vi "Main.vi"(11 "Module Admin":refnum<class "Delacor_lib_QMH_Module Admin.lvclass">) -> ()   [LabVIEW 2020, in "Stock.lvlib"]
doc: "This template is based off of the Queued Message Handler design pattern and the Queued Message Handler project template that ships with LabVIEW.\n\nThe main difference is that the queue is private to this module and communication between modules is performed via Broadcast and Request events.\n\nRequest events are wrapped in public API methods and are handled in the Event Handling Loop (EHL) of this VI. Any module can register for Broadcast events sent by this module. The EHL generates messages based on user interface actions.\n\nThe Message Handling Loop (MHL) processes messages generated by the EHL, or by other messages. The messages are string values, so new messages can be added easily to the Message Cases case structure in the MHL. Each message cluster can also provide an optional value for Message Data, which is a variant that can be converted to whatever message-specific data is required.\n_____\nBased on Delacor QMH Project Template 5.0.0.82."
uses:
  Stock.lvlib
  <vilib>/Delacor/Delacor QMH/Libraries/Module Admin_class/Delacor_lib_QMH_Module Admin.lvclass
  Module Data--cluster.ctl
  <vilib>/Delacor/Delacor QMH/Libraries/Message Queue_class/Delacor_lib_QMH_Message Queue.lvclass/Delacor_lib_QMH_Message Queue.ctl
  Stop Argument--cluster.ctl
  <vilib>/Delacor/Delacor QMH/Libraries/Module Admin_class/Delacor_lib_QMH_Module Admin.lvclass/Delacor_lib_QMH_Module Admin.ctl
  Check Product Availability Argument--cluster.ctl
  Check Product Availability (Reply Payload)--cluster.ctl
  Extract Product Argument--cluster.ctl
  <vilib>/Utility/miscctls.llb/LVPointTypeDef.ctl
  <vilib>/Delacor/Delacor QMH/Libraries/Message Queue_class/Delacor_lib_QMH_Enqueue Message (Single).vi
  <vilib>/Delacor/Delacor QMH/Libraries/Module Admin_class/Delacor_lib_QMH_Get External Launch.vi
  <vilib>/Utility/error.llb/Error Cluster From Error Code.vi
  <vilib>/ErrorRing/Error Ring.xnode
  <vilib>/Delacor/Delacor QMH/Libraries/Message Queue_class/Delacor_lib_QMH_Message Queue.lvclass
panel:
  in  "Products":T1(array[cluster])=[{"Product name"="Coke", "Quantity"=10.0, "Price"=5.0}, {"Product name"="Sprite", "Quantity"=10.0, "Price"=4.5}, {"Product name"="Orange Juice", "Quantity"=10.0, "Price"=6.0}, {"Product name"="Regular water", "Quantity"=10.0, "Price"=3.5}, {"Product name"="Sparking water", "Quantity"=10.0, "Price"=3.5}]
  in  "Simulate MHL Error":bool
  in  "Simulate EHL Error":bool
  out "error out":errorcluster
  out "Status":string
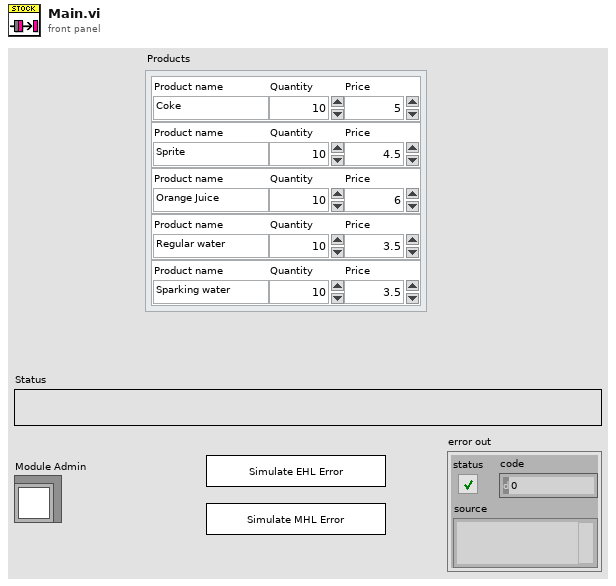
[diagram p1: front panel]
types:
  T1 = cluster{"Product name":string, "Quantity":dbl, "Price":dbl}[]
  T2 = typedef "Stock.lvlib/Request Events--cluster.ctl" = cluster{"Stop Module":refnum<user-event>, "Show Panel":refnum<user-event>, "Hide Panel":refnum<user-event>, "Get Module Execution Status":refnum<user-event>, "Show Diagram":refnum<user-event>, "Check Product Availability":refnum<user-event>, "Extract Product":refnum<user-event>}
  T3 = typedef "Stock.lvlib/Module Data--cluster.ctl" = cluster{"Status":string, "Map":map{string, cluster{"Product name":string, "Quantity":dbl, "Price":dbl}}}
  T4 = enum32{"invalid lock state", "Not Locked", "Locked (No Password)", "Password-protected"}
  T5 = typedef "Stock.lvlib/Stop Argument--cluster.ctl" = cluster{"Origin":string, "Exit via Stop Module Req?":bool, "Wait for Module to stop?":bool}
  T6 = typedef "Stock.lvlib/Check Product Availability Argument--cluster.ctl" = cluster{"Product name":string, "Wait Notifier":refnum<notifier>, "wait for reply":bool}
  T7 = typedef "Stock.lvlib/Extract Product Argument--cluster.ctl" = cluster{"Product name":string}
  T8 = typedef "LVPointTypeDef.ctl" = cluster{"Horizontal":i16, "Vertical":i16}
  T9 = enum32{"Invalid", "Standard", "Closed", "Hidden", "Minimized", "Maximized"}
  T10 = typedef "Stock.lvlib/Check Product Availability (Reply Payload)--cluster.ctl" = cluster{"Product in stock":bool, "Check Product Availability_error":errorcluster}
  T11 = map{string, cluster{"Product name":string, "Quantity":dbl, "Price":dbl}}
  T12 = cluster{"Product name":string, "Quantity":dbl, "Price":dbl}
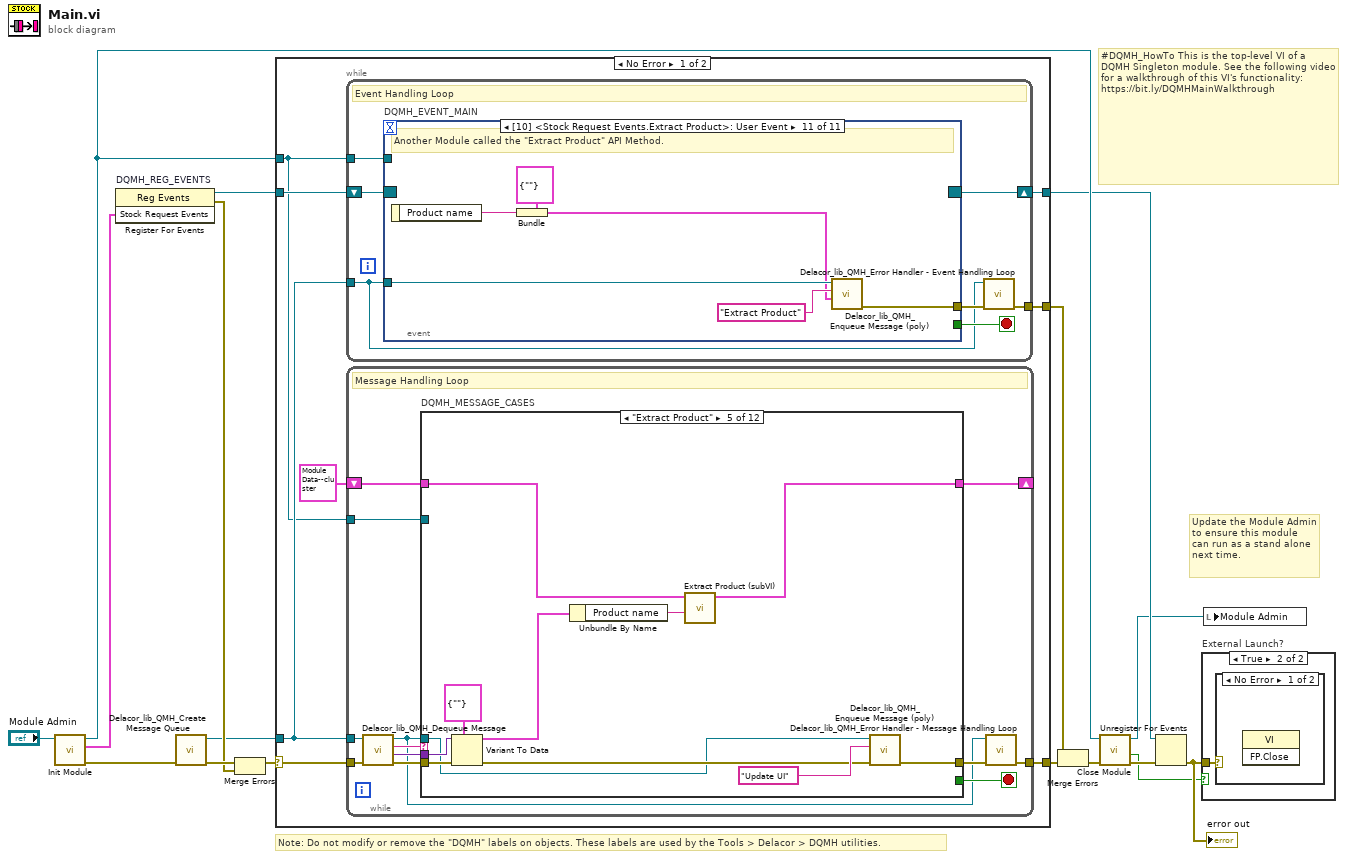
[diagram p0: block diagram]
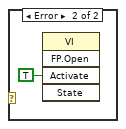
[diagram p3: hidden frame]
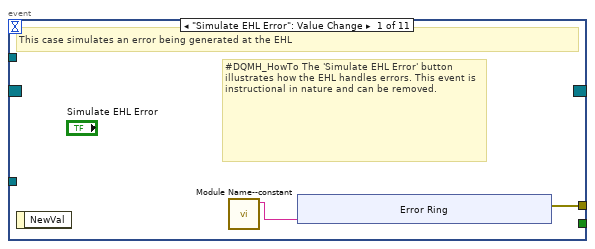
[diagram p4: hidden frame]
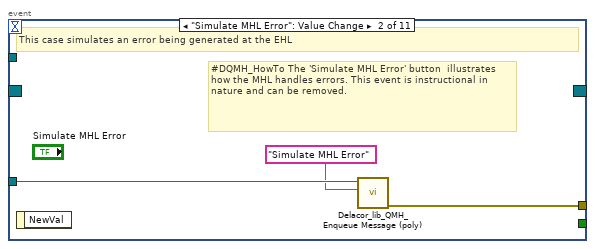
[diagram p5: hidden frame]
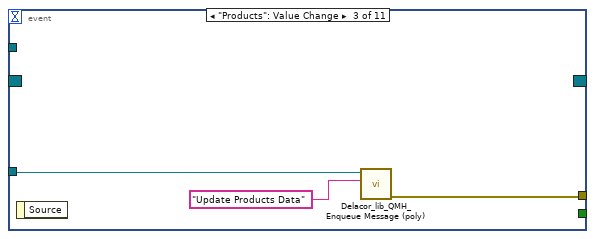
[diagram p6: hidden frame]
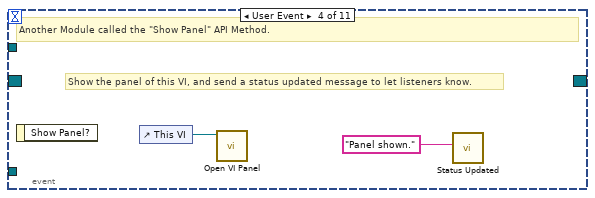
[diagram p7: hidden frame]
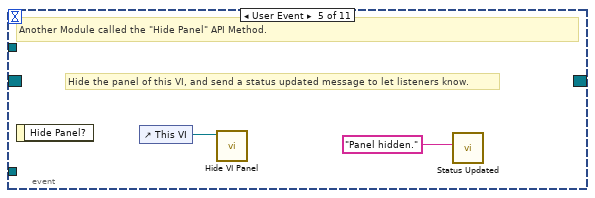
[diagram p8: hidden frame]
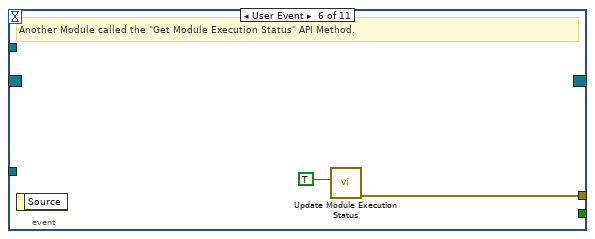
[diagram p9: hidden frame]
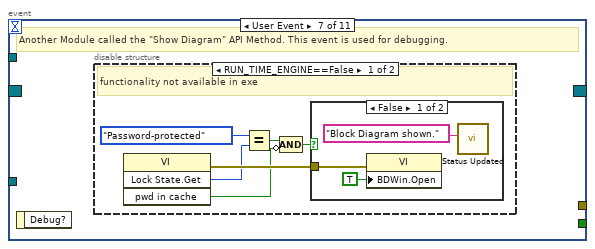
[diagram p10: hidden frame]
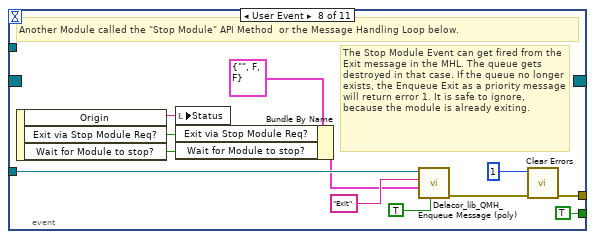
[diagram p13: hidden frame]
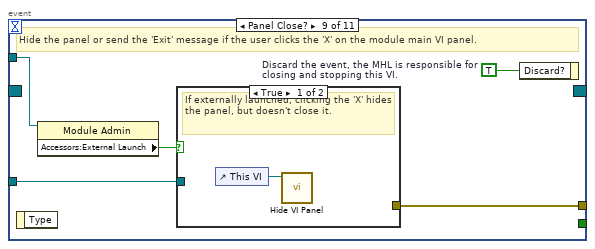
[diagram p14: hidden frame]
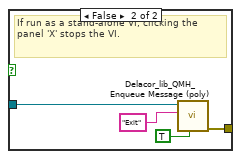
[diagram p15: hidden frame]
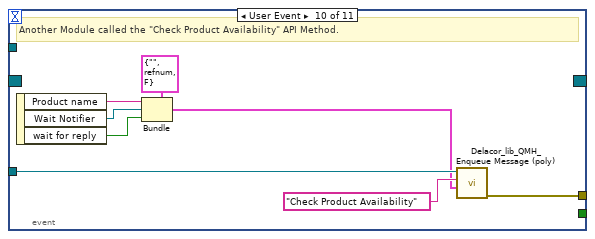
[diagram p16: hidden frame]
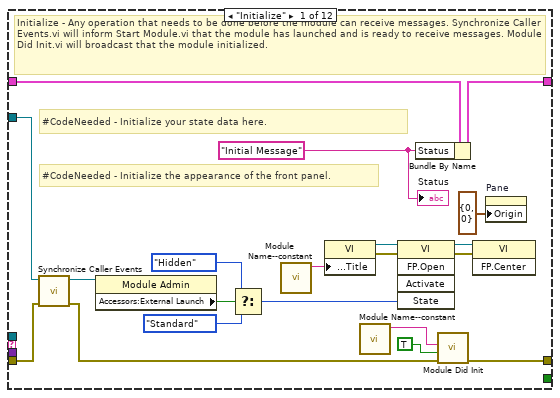
[diagram p17: hidden frame]
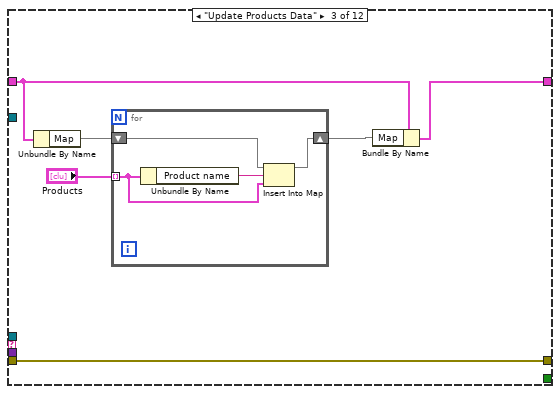
[diagram p19: hidden frame]
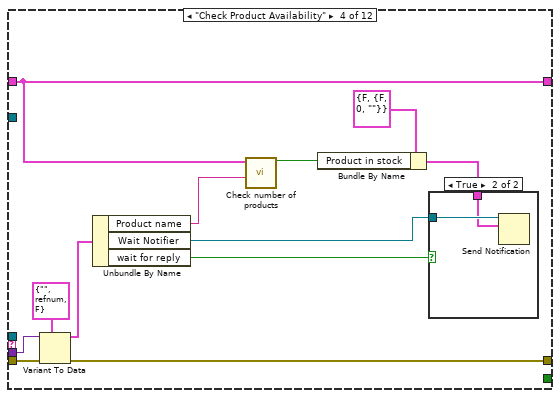
[diagram p20: hidden frame]
diagram:
  # "#DQMH_HowTo This is the top-level VI of a DQMH Singleton module. See the following video for a walkthrough of this VI's functionality: https://bit.ly/DQMHMainWalkthrough"
  # "Note: Do not modify or remove the \"DQMH\" labels on objects. These labels are used by the Tools > Delacor > DQMH utilities."
  # "Update the Module Admin to ensure this module can run as a stand alone next time."
  n1 = call "Init Module.vi"("Singleton Module Admin in"="Module Admin") -> ("error out"=w16:errorcluster, "Stock Request Events"=w5:T2, "Singleton Module Admin out"=w8:refnum<class "Delacor_lib_QMH_Module Admin.lvclass">)  [unwired: 8 in]
  n2 = register-events "DQMH_REG_EVENTS"(w5) -> (reference out=w6:refnum<event-registration>, error out=w9:errorcluster)  [unwired: 2 in]
  n3 = call <vilib>:"Delacor_lib_QMH_Create Message Queue.vi"("error in (no error)"=w16) -> ("error out"=w11:errorcluster, "Message Queue"=w4:refnum<class "Delacor_lib_QMH_Message Queue.lvclass">)  [unwired: 9 in]
  n4 = Merge Errors(w11, w9) -> (w10:errorcluster)
  n5 = case shown="No Error" w10 {
    selector: w10 -> [w23 w239]
    tunnel: [w25 w238] -> w17
    tunnel: [w22 w244] -> w7
    tunnel: w6 -> [w20 w244]
    tunnel: w4 -> [w19 w237]
    tunnel: [w24 _] -> w14
    tunnel: w8 -> [w18 w240]
    frame No Error {
      n6 = while {
        tunnel: w19 -> [w26]
        shift-right: [w29] -> w22
        shift-left: w20 -> [w30]
        tunnel: [w31] -> w24
        tunnel: w18 -> [w27]
        stop <- w28 stop-if-true
        # "Event Handling Loop"
        n7 = event "DQMH_EVENT_MAIN" shown="[10] <Stock Request Events.Extract Product>: User Event" {
          selector: w30 -> [_ _ _ _ _ _ _ _ _ _ _]
          dyn-events: [_ _ _ _ _ _ _ _ _ _ _] -> w29
          timeout: _ -> [_ _ _ _ _ _ _ _ _ _ _]
          tunnel: [_ _ _ _ _ _ _ TRUE ("Discard?") _ _ _] -> w28
          tunnel: w26 -> [_ w43 w46 _ _ _ _ w70 w77 w92 w98]
          tunnel: [w34 w44 w45 _ _ w53 _ w73 w79 w85 w93] -> w32
          tunnel: w27 -> [_ _ _ _ _ _ _ _ w76 _ _]
          event "Simulate EHL Error": Value Change {
            # "#DQMH_HowTo The 'Simulate EHL Error' button  illustrates how the EHL handles errors. This event is instructional in nature and can be removed."
            # "This case simulates an error being generated at the EHL"
            n8 = event-data() -> ()  [unwired: 1 in, 1 out]
            n9 = call "Module Name--constant.vi"() -> ("Module Name"=w33:string)  [unwired: 11 in]
            n10 = xnode "Error Ring"("parameter 0"=w33) -> ("error out"=w34:errorcluster)
          }
          event "Simulate MHL Error": Value Change {
            # "#DQMH_HowTo The 'Simulate MHL Error' button  illustrates how the MHL handles errors. This event is instructional in nature and can be removed."
            # "This case simulates an error being generated at the EHL"
            n11 = event-data() -> ()  [unwired: 1 in, 1 out]
            n12 = call-poly <vilib>:"Delacor_lib_QMH_Enqueue Message (poly).vi"("Message"="Simulate MHL Error", "Message Queue in"=w43) -> ("error out"=w44:errorcluster)  [unwired: 8 in, 1 out]
          }
          event "Products": Value Change {
            n13 = event-data() -> ()  [unwired: 1 in, 1 out]
            n14 = call-poly <vilib>:"Delacor_lib_QMH_Enqueue Message (poly).vi"("Message"="Update Products Data", "Message Queue in"=w46) -> ("error out"=w45:errorcluster)  [unwired: 8 in, 1 out]
          }
          event User Event {
            # "Show the panel of this VI, and send a status updated message to let listeners know."
            # "Another Module called the \"Show Panel\" API Method."
            n15 = event-data() -> ()  [unwired: 1 in, 1 out]
            n16 = control-ref of="This VI"() -> (w49:refnum<vi>)
            n17 = call "Open VI Panel.vi"("VI"=w49) -> ()  [unwired: 10 in, 1 out]
            n18 = call "Status Updated.vi"("Status"="Panel shown." ("format string")) -> ()  [unwired: 10 in, 1 out]
          }
          event User Event {
            # "Hide the panel of this VI, and send a status updated message to let listeners know."
            # "Another Module called the \"Hide Panel\" API Method."
            n19 = event-data() -> ()  [unwired: 1 in, 1 out]
            n20 = control-ref of="This VI"() -> (w51:refnum<vi>)
            n21 = call "Hide VI Panel.vi"("VI"=w51) -> ()  [unwired: 10 in, 1 out]
            n22 = call "Status Updated.vi"("Status"="Panel hidden." ("format string")) -> ()  [unwired: 10 in, 1 out]
          }
          event User Event {
            # "Another Module called the \"Get Module Execution Status\" API Method."
            n23 = event-data() -> ()  [unwired: 1 in, 1 out]
            n24 = call "Update Module Execution Status.vi"("Running?"=TRUE) -> ("error out"=w53:errorcluster)  [unwired: 10 in]
          }
          event User Event {
            # "Another Module called the \"Show Diagram\" API Method. This event is used for debugging."
            n25 = event-data() -> ()  [unwired: 1 in, 1 out]
            n26 = disable-structure shown="RUN_TIME_ENGINE==False" {
              frame condition #0 (active) {
                # "functionality not available in exe"
                n27 = invoke class="VI" method="Lock State.Get"() -> (error out=w59:errorcluster, "Get Lock State"=w58:T4, "pwd in cache"=w55:bool)  [unwired: 4 in, 1 out]
                n28 = Equal?(x=T4."Password-protected", y=w58) -> (x = y?=w56:bool)
                n29 = Compound Arithmetic op=AND(w56, invert w55) -> (w54:bool)
                n30 = case shown="False" w54 {
                  tunnel: w59 -> [w62 _]
                  frame False {
                    n31 = property class="VI"(error in=w62, "BDWin.Open"=TRUE ("Block Diagram Window:Open")) -> ()  [unwired: 1 in, 2 out]
                    n32 = call "Status Updated.vi"("Status"="Block Diagram shown." ("format string")) -> ()  [unwired: 10 in, 1 out]
                  }
                  frame True {
                    # "Password-protected VI, and the password is not in the cache. Do not show the diagram."
                  }
                }
              }
              frame condition #1 {
              }
            }
          }
          event User Event {
            # "The Stop Module Event can get fired from the Exit message in the MHL. The queue gets destroyed in that case. If the queue no longer exists, the Enqueue Exit as a priority message will return error 1. It is safe to ignore, because the module is already exiting."
            # "Another Module called the \"Stop Module\" API Method  or the Message Handling Loop below."
            n33 = event-data() -> ("Origin"=w69:string, "Exit via Stop Module Req?"=w65:bool, "Wait for Module to stop?"=w64:bool)  [unwired: 1 in]
            n34 = local write "Status"(w69) -> ()
            n35 = Bundle By Name(cluster=T5 {"Origin"="", "Exit via Stop Module Req?"=FALSE, "Wait for Module to stop?"=FALSE} ("Stop Argument"), "Exit via Stop Module Req?"=w65, "Wait for Module to stop?"=w64) -> (w63:T5)
            n36 = call-poly <vilib>:"Delacor_lib_QMH_Enqueue Message (poly).vi"("Priority Message? (F)"=TRUE, "Message Data"=w63, "Message"="Exit", "Message Queue in"=w70) -> ("error out"=w74:errorcluster)  [unwired: 6 in, 1 out]
            n37 = call <vilib>:"Clear Errors.vi"("error in (no error)"=w74, "specific error code to clear (0: all)"=1) -> ("error out"=w73:errorcluster)  [unwired: 4 in, 1 out]
          }
          event Panel Close? {
            w78 = TRUE  # Discard the event, the MHL is responsible for closing and stopping this VI.
            # "Hide the panel or send the 'Exit' message if the user clicks the 'X' on the module main VI panel."
            n38 = event-data() -> ()  [unwired: 1 in, 1 out]
            n39 = property class="Module Admin"(reference=w76) -> ("Accessors:External Launch"=w75:bool)  [unwired: 1 in, 2 out]
            n40 = case shown="True" w75 {
              tunnel: w77 -> [_ w83]
              tunnel: [_ w84] -> w79
              frame True {
                # "If externally launched, clicking the 'X' hides the panel, but doesn't close it."
                n41 = control-ref of="This VI"() -> (w80:refnum<vi>)
                n42 = call "Hide VI Panel.vi"("VI"=w80) -> ()  [unwired: 10 in, 1 out]
              }
              frame False {
                # "If run as a stand-alone VI, clicking the panel 'X' stops the VI."
                n43 = call-poly <vilib>:"Delacor_lib_QMH_Enqueue Message (poly).vi"("Priority Message? (F)"=TRUE, "Message"="Exit", "Message Queue in"=w83) -> ("error out"=w84:errorcluster)  [unwired: 7 in, 1 out]
              }
            }
            n44 = event-data("Discard?"=w78) -> ()  [unwired: 1 in, 1 out]
          }
          event User Event {
            # "Another Module called the \"Check Product Availability\" API Method."
            n45 = event-data() -> ("Product name"=w88:string, "Wait Notifier"=w87:refnum<notifier>, "wait for reply"=w86:bool)  [unwired: 1 in]
            n46 = Bundle(cluster=T6 {"Product name"="", "Wait Notifier"=refnum, "wait for reply"=FALSE} ("Check Product Availability Argument"), "Product name"=w88, "Wait Notifier"=w87, "wait for reply"=w86) -> (w89:T6)
            n47 = call-poly <vilib>:"Delacor_lib_QMH_Enqueue Message (poly).vi"("Message Data"=w89, "Message"="Check Product Availability", "Message Queue in"=w92) -> ("error out"=w85:errorcluster)  [unwired: 7 in, 1 out]
          }
          event User Event {
            # "Another Module called the \"Extract Product\" API Method."
            n48 = event-data() -> ("Product name"=w94:string)  [unwired: 1 in]
            n49 = Bundle(cluster=T7 {"Product name"=""} ("Extract Product Argument"), "Product name"=w94) -> (w95:T7)
            n50 = call-poly <vilib>:"Delacor_lib_QMH_Enqueue Message (poly).vi"("Message Data"=w95, "Message"="Extract Product", "Message Queue in"=w98) -> ("error out"=w93:errorcluster)  [unwired: 7 in, 1 out]
          }
        }
        n51 = call-dynamic "Delacor_lib_QMH_Error Handler - Event Handling Loop.vi"("error in (no error)"=w32, "Message Queue in"=w26) -> ("dup error in"=w31:errorcluster)  [unwired: 8 in, 1 out]
      }
      n52 = while {
        tunnel: w19 -> [w101]
        shift-right: [w105] -> _
        shift-left: T3 {"Status"="", "Map"={}} ("Data Cluster") -> [w106]
        tunnel: w23 -> [w109]
        tunnel: [w107] -> w25
        tunnel: w18 -> [w99]
        stop <- w104 stop-if-true
        # "Message Handling Loop"
        n53 = call-dynamic "Delacor_lib_QMH_Dequeue Message.vi"("error in (no error)"=w109, "Message Queue in"=w101) -> ("error out"=w108:errorcluster, "Message Data"=w102:variant, "Message"=w103:string, "Message Queue out"=w100:refnum<class "Delacor_lib_QMH_Message Queue.lvclass">)  [unwired: 6 in]
        n54 = case "DQMH_MESSAGE_CASES" shown="\"Extract Product\"" w103 {
          selector: w103 -> [_ _ _ _ _ _ _ _ _ _ _ w224]
          tunnel: w100 -> [_ _ _ _ w157 _ _ _ _ w194 w216 _]
          tunnel: w108 -> [w128 w132 w138 w154 w167 w171 w176 w178 w183 w201 w222 w226]
          tunnel: [w126 w132 w138 w143 w158 w171 w175 w178 w182 w197 w219 w227] -> w110
          tunnel: w106 -> [w117 w131 w134 w146 w163 w170 w174 w177 w180 w196 w215 w225]
          tunnel: [w116 w131 w137 w146 w162 w170 w174 w177 w180 w196 w215 w225] -> w105
          tunnel: [_ _ _ _ _ _ _ _ _ _ w214 _] -> w104
          tunnel: w102 -> [_ _ _ w153 w166 _ _ _ _ w195 w213 _]
          tunnel: w99 -> [w118 _ _ _ _ _ _ _ _ w193 w208 _]
          frame "Initialize" {
            w111 = "Initial Message" ("Initial Message")
            # "#CodeNeeded - Initialize the appearance of the front panel."
            # "#CodeNeeded - Initialize your state data here."
            # "Initialize - Any operation that needs to be done before the module can receive messages. Synchronize Caller Events.vi will inform Start Module.vi that the module has launched and is ready to receive messages. Module Did Init.vi will broadcast that the module initialized."
            n55 = call "Synchronize Caller Events.vi"("error in (no error)"=w128, "Singleton Module Admin in"=w118) -> ("error out"=w127:errorcluster, "Singleton Module Admin out"=w113:refnum<class "Delacor_lib_QMH_Module Admin.lvclass">)  [unwired: 8 in]
            n56 = property class="Module Admin"(reference=w113) -> ("Accessors:External Launch"=w122:bool)  [unwired: 1 in, 2 out]
            n57 = Select(t=T9."Hidden" ("State"), s=w122, f=T9."Standard" ("State")) -> (s? t:f=w119:T9)
            n58 = call "Module Name--constant.vi"() -> ("Module Name"=w125:string)  [unwired: 11 in]
            n59 = property class="VI"("Front Panel.Title"=w125) -> (reference out=w124:refnum<vi>, error out=w130:errorcluster)  [unwired: 2 in]
            n60 = call "Module Name--constant.vi"() -> ("Module Name"=w114:string)  [unwired: 11 in]
            n61 = invoke class="VI" method="FP.Open"(reference=w124, error in=w130, "State"=w119) -> (reference out=w123:refnum<vi>, error out=w129:errorcluster)  [unwired: 2 in, 3 out]
            n62 = Bundle By Name(cluster=w117, "Status"=w111) -> (w116:T3)
            n63 = call "Module Did Init.vi"("error in (no error)"=w127, "Initialized?"=TRUE, "Origin"=w114) -> ("error out"=w126:errorcluster)  [unwired: 8 in]
            n64 = invoke class="VI" method="FP.Center"(reference=w123, error in=w129) -> ()  [unwired: 1 in, 3 out]
            n65 = property on="Pane" class="Pane"("Origin"=T8 {"Horizontal"=0, "Vertical"=0}) -> ()  [unwired: 2 in, 2 out]
            "Status" <- w111
          }
          frame "--- Module Specific ---" {
            # "Separator -- The following cases handle messages specific to this Module."
          }
          frame "Update Products Data" {
            n66 = Unbundle By Name(w134) -> ("Map"=w135:T11)
            n67 = for {
              tunnel: "Products" -> [w141] mode=indexing
              shift-right: [w139] -> w133
              shift-left: w135 -> [w140]
              n68 = Unbundle By Name(w141) -> ("Product name"=w142:string)
              n69 = Insert Into Map(map in=w140, key=w142, value=w141) -> (map out=w139:T11)  [unwired: 2 out]
            }
            n70 = Bundle By Name(cluster=w134, "Map"=w133) -> (w137:T3)
          }
          frame "Check Product Availability" {
            n71 = Variant To Data(error in=w154, type=T6 {"Product name"="", "Wait Notifier"=refnum, "wait for reply"=FALSE} ("Check Product Availability Argument"), Variant=w153) -> (data=w151:T6, error out=w143:errorcluster)
            n72 = Unbundle By Name(w151) -> ("Product name"=w145:string, "Wait Notifier"=w150:refnum<notifier>, "wait for reply"=w149:bool)
            n73 = call "Check number of products.vi"("Product name"=w145, "Data Cluster"=w146) -> ("Product Available"=w144:bool)  [unwired: 9 in]
            n74 = Bundle By Name(cluster=T10 {"Product in stock"=FALSE, "Check Product Availability_error"={"status"=FALSE, "code"=0, "source"=""}} ("Check Product Availability (Reply Payload)"), "Product in stock"=w144) -> (w148:T10)
            n75 = case shown="True" w149 {
              tunnel: w150 -> [_ w156]
              tunnel: w148 -> [_ w155]
              frame False {
              }
              frame True {
                n76 = Send Notification(notification=w155, notifier=w156) -> ()  [unwired: 1 in, 2 out]
              }
            }
          }
          frame "Extract Product" {
            n77 = Variant To Data(error in=w167, type=T7 {"Product name"=""} ("Extract Product Argument"), Variant=w166) -> (data=w164:T7, error out=w159:errorcluster)
            n78 = Unbundle By Name(w164) -> ("Product name"=w161:string)
            n79 = call "Extract Product (subVI).vi"("Product name"=w161, "Data Cluster"=w163) -> ("Data cluster output"=w162:T3)  [unwired: 9 in]
            n80 = call-poly <vilib>:"Delacor_lib_QMH_Enqueue Message (poly).vi"("error in (no error)"=w159, "Message"="Update UI", "Message Queue in"=w157) -> ("error out"=w158:errorcluster)  [unwired: 7 in, 1 out]
          }
          frame "Update UI" {
            n81 = Unbundle By Name(w170) -> ("Map"=w169:T11)
            n82 = for {
              tunnel: w169 -> [w173] mode=indexing
              tunnel: [w172] -> w168 mode=indexing
              n83 = Unbundle By Name(w173) -> ("Cluster"=w172:T12)
            }
            n84 = local write "Products"(w168) -> ()
          }
          frame "---Copy This Frame---" {
            # "Duplicate this frame when creating new messages.  Change this comment in the duplicated frame to describe this message."
            n85 = Merge Errors(w176) -> (w175:errorcluster)
          }
          frame "--- Exit and Error Handling---" {
            # "Separator - The following cases handle errors and exit messages."
          }
          frame "Simulate MHL Error" {
            # "#DQMH_HowTo The 'Simulate MHL Error' button  illustrates how the MHL handles errors. This event is instructional in nature and can be removed."
            # "Simulate an error occurring at the MHL"
            n86 = call "Module Name--constant.vi"() -> ("Module Name"=w179:string)  [unwired: 11 in]
            n87 = xnode "Error Ring"("parameter 0"=w179) -> ("error out"=w181:errorcluster)
            n88 = Merge Errors(w183, w181) -> (w182:errorcluster)
          }
          frame "Error" {
            # "#CodeRecommended - If you ever change the name of this \"Error\" message, you'll need to update the name in the Check Loop Error.vi as well."
            # "#CodeRecommended - If the module is running in standalone mode (External Launch = FALSE), this code will pop up an error dialog and call the 'Exit' message if an error occurs. Add more fine-grained error handling here."
            # "Error - Check the error message data and respond accordingly. This message is sent by the \"Error Handler\" VIs at the end of each loop in this application."
            n89 = property class="Module Admin"(reference=w193) -> ("Accessors:External Launch"=w192:bool)  [unwired: 1 in, 2 out]
            n90 = Variant To Data(error in=w201, type=errorcluster {"status"=FALSE, "code"=0, "source"=""} ("error constant"), Variant=w195) -> (data=w202:errorcluster, error out=w199:errorcluster)
            n91 = call "Module Name--constant.vi"() -> ("Module Name"=w191:string)  [unwired: 11 in]
            n92 = call "Error Reported.vi"("Additional Information"=w191, "Error"=w202) -> ()  [unwired: 9 in, 1 out]
            n93 = case shown="False" w192 {
              tunnel: [w207 _] -> w198
              tunnel: w194 -> [w205 _]
              tunnel: w202 -> [w206 _]
              frame False {
                # "If the module is running standalone, then pop up an error dialog and call the \"Exit\" message."
                n94 = call <vilib>:"Simple Error Handler.vi"("error in (no error)"=w206) -> ()  [unwired: 4 in, 5 out]
                n95 = call-poly <vilib>:"Delacor_lib_QMH_Enqueue Message (poly).vi"("Priority Message? (F)"=TRUE, "Message"="Exit", "Message Queue in"=w205) -> ("error out"=w207:errorcluster)  [unwired: 7 in, 1 out]
              }
              frame True {
                # "If the module was launched externally, calling the Error Reported broadcast VI is the only action performed by the \"Error\" message. The module's caller can then process the error appropriately."
              }
            }
            n96 = Merge Errors(w199, w198) -> (w197:errorcluster)
            n97 = local write "error out"(w197) -> ()
          }
          frame "Exit" {
            w212 = 91  # 91: not all Exit messages will have an argument
            w214 = TRUE  # Stop the VI
            # "Release the message queue reference"
            # "#CodeNeeded - Add any required cleanup code here"
            # "Exit - Exit the application."
            n98 = Variant To Data(error in=w222, type=T5 {"Origin"="", "Exit via Stop Module Req?"=FALSE, "Wait for Module to stop?"=FALSE} ("Stop Argument"), Variant=w213) -> (data=w210:T5, error out=w218:errorcluster)
            n99 = call <vilib>:"Clear Errors.vi"("error in (no error)"=w218, "specific error code to clear (0: all)"=w212) -> ("error out"=w221:errorcluster)  [unwired: 4 in, 1 out]
            n100 = control-ref of="This VI"() -> (w209:refnum<vi>)
            n101 = call-dynamic "Delacor_lib_QMH_Release Message Queue.vi"("error in (no error)"=w221, "Message Queue"=w216) -> ("error out"=w220:errorcluster)  [unwired: 9 in]
            n102 = call "Handle Exit.vi"("Stop Argument"=w210, "Admin in"=w208, "VI reference"=w209) -> ("error out"=w217:errorcluster)  [unwired: 7 in, 1 out]
            n103 = Merge Errors(w220, w217) -> (w219:errorcluster)
          }
          frame Default {
            # "'Default' case only runs if there is a message that isn't defined in any of the other cases.  Output a programming error."
            n104 = call "Module Name--constant.vi"() -> ("Module Name"=w223:string)  [unwired: 11 in]
            n105 = xnode "Error Ring"("parameter 0"=w224, "parameter 1"=w223) -> ("error out"=w228:errorcluster)
            n106 = Merge Errors(w226, w228) -> (w227:errorcluster)
          }
        }
        n107 = call-dynamic "Delacor_lib_QMH_Error Handler - Message Handling Loop.vi"("error in (no error)"=w110, "Message Queue in"=w100) -> ("dup error in"=w107:errorcluster)  [unwired: 8 in, 1 out]
      }
    }
    frame Error {
      # "Synchronize Caller Events.vi will inform Start Module.vi that the module has launched and will let the code calling Start Module.vi register for broadcasts and would permit the caller receive the broadcast that an error occurred at launch time."
      n108 = call-dynamic "Delacor_lib_QMH_Release Message Queue.vi"("error in (no error)"=w239, "Message Queue"=w237) -> ("error out"=w238:errorcluster)  [unwired: 9 in]
      n109 = call "Synchronize Caller Events.vi"("Singleton Module Admin in"=w240) -> ("error out"=w245:errorcluster)  [unwired: 9 in, 1 out]
      n110 = call "Module Name--constant.vi"() -> ("Module Name"=w243:string)  [unwired: 11 in]
      n111 = Format Into String(format string="An error occurred during initialization. %s is no longer running.", w243) -> (resulting string=w241:string)  [unwired: 2 in, 1 out]
      n112 = Merge Errors(w238, w245) -> (w246:errorcluster)
      n113 = call "Error Reported.vi"("Additional Information"=w241, "Error"=w246) -> ()  [unwired: 9 in, 1 out]
    }
  }
  n114 = Merge Errors(w14, w17) -> (w13:errorcluster)
  n115 = call "Close Module.vi"("error in (no error)"=w13, "Module Admin in"=w8) -> ("error out"=w15:errorcluster, "External Launch"=w1:bool, "Module Admin out"=w2:refnum<class "Delacor_lib_QMH_Module Admin.lvclass">)  [unwired: 7 in]
  n116 = Unregister For Events(event registration refnum=w7, error in=w15) -> (error out=w12:errorcluster)
  "error out" <- w12
  n117 = case "External Launch?" shown="True" w1 {
    tunnel: w12 -> [_ w247]
    frame False {
    }
    frame True {
      n118 = case shown="No Error" w247 {
        frame No Error {
          n119 = invoke class="VI" method="FP.Close"() -> ()  [unwired: 3 in, 3 out]
        }
        frame Error {
          n120 = invoke class="VI" method="FP.Open"("Activate"=TRUE ("Activate?")) -> ()  [unwired: 4 in, 5 out]
        }
      }
    }
  }
  n121 = local write "Module Admin"(w2) -> ()
